vi "Dashboard Main.vi.REMOTE.11652.vi"() -> ()   [LabVIEW 2014]
uses:
  AutonModes.ctl
  <vilib>/event_ctls.llb/eventvkey.ctl
  <vilib>/Utility/error.llb/DialogType.ctl
  <vilib>/Rock Robotics/WPI/Dashboard/WPI_DashboardLogging Global.vi
  <vilib>/Rock Robotics/Network Tables/SD Write String.vi
  <vilib>/Rock Robotics/Network Tables/SD Read String.vi
  <vilib>/Utility/config.llb/Write Key (String).vi
  <vilib>/Utility/config.llb/Write Key (I32).vi
  <vilib>/Utility/config.llb/NI_LVConfig.lvlib
panel:
  in  "TCP":refnum<k5>
  in  "Rec Mode":enum32{"Stop", "Record", "Playback"}(radio)
  in  "Vision":u16(ring) items=["Camera Off", "USB Camera SW", "USB Camera HW", "IP Camera"]
  out "Camera IP":string
  out "Image Message":string="Timeout in Camera Communications"
  in  "Dashboard Tab":T1(tab)
  in  "Camera Settings":T2={"Frame Rate"=30, "Compression"=30, "Size"=1} {"Frame Rate" scale=1.0..30.0; "Size" items=["640x480", "320x240", "160x120"]}
  out "MotorChart R":cluster{"Numeric":dbl, "Numeric":dbl}(graph)
  out "MotorChart L":T3(graph)
  out "MotorSliders R":cluster{"MotorSlide1":dbl, "MotorSlide2":dbl} {"MotorSlide2" scale=-1.0..1.0 scale format="%#_2e"; "MotorSlide1" scale=-1.0..1.0 scale format="%#_2e"}
  out "MotorSliders L":T4 {"MotorSlide4 2" scale=0.0..14.0 scale format="%#_2e"; "MotorSlide2" scale=-1.0..1.0 scale format="%#_2e"; "MotorSlide1" scale=-1.0..1.0 scale format="%#_2e"}
  out "Gyro":dbl(knob) scale=0.0..360.0
  out "JS1 Z":dbl(slide) scale=-1.0..1.0 scale format="%#_2e"
  out "JS1 Graph":cluster{"X":dbl, "Y":dbl}[](graph)
  out "JS1 Buttons":T5
  out "JS2 Z":dbl(slide) scale=-1.0..1.0 scale format="%#_2e"
  out "JS2 Graph":cluster{"X":dbl, "Y":dbl}[](graph)
  out "JS2 Buttons":T5
  out "Mode":T6(ring)=enum."Auto Disabled"
  in  "DB Camera Config":bool
  out "fps":dbl format="%#.1g"
  out "Mbps":dbl format="%#.1g"
  out "Mbps 2":bool
  in  "Open Config File":bool
  in  "Auton Mode":T7
  in  "Path to Auton Configs":path=path "C:/AutoConfig"
  out "Current Overdraw":bool
  out "Current":T8(graph)
  in  "DB/String 9":string
  in  "DB/String 8":string
  in  "DB/String 7":string
  in  "DB/String 6":string
  in  "DB/String 5":string
  in  "DB/String 4":string
  in  "DB/String 3":string
  in  "DB/String 2":string
  in  "DB/String 1":string
  in  "DB/String 0":string
  in  "DB/Slider 0":dbl(slide) scale=0.0..5.0
  in  "DB/Slider 1":dbl(slide) scale=0.0..5.0
  in  "DB/Slider 2":dbl(slide) scale=0.0..5.0
  in  "DB/Slider 3":dbl(slide) scale=0.0..5.0
  out "DB/LED 3":bool
  out "DB/LED 2":bool
  out "DB/LED 1":bool
  out "DB/LED 0":bool
  in  "DB/Button 3":bool
  in  "DB/Button 2":bool
  in  "DB/Button 1":bool
  in  "DB/Button 0":bool caption="New Name"
  in  "Test Slider":dbl(slide) scale=0.0..100.0 scale format="%#_3g"
  in  "On/Off":bool caption="Solenoid"
  in  "Test Name":u16(ring) items=["Select the test to run...", "Example Test", "-------------------------------", "List of tests is built in robot code.", "Replace with your own automated tests."]
  in  "Test Tree":string(tree)
  in  "Motor":cluster{"Value":dbl, "Enable":bool} {"Value" scale=-1.0..1.0 scale format="%#_3g"}
  out "Progress":T9 {"Test Progress" scale=0.0..100.0}
  in  "Rev/Fwd":cluster{"Forward":bool, "Reverse":bool}
  in  "Test Ring":u16(ring) items=["Monochrome", "Color"]
  in  "Listbox":i32(listbox)
  out "Tree":string(tree)
  out "Camera Image":T10(plugin-control)
  out "Boolean":bool
  # "Left"
  # "Front"
  # "Right"
  # "Battery"
  # "This tab is a great place for autonomous settings and robot-specific values.\nPlace controls and indicators inside this tab and match name to\nDashboard Variables on robot. You can also delete this comment."
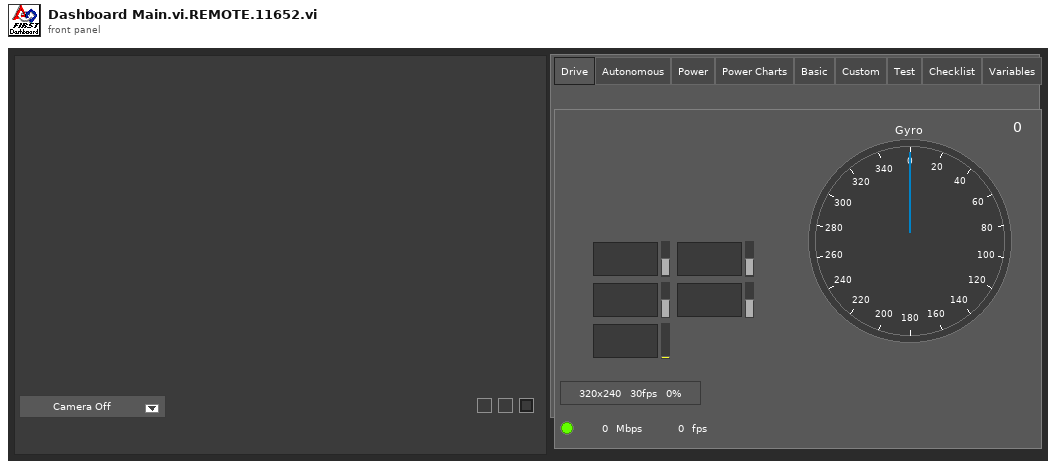
[diagram p1: front panel]
types:
  T1 = enum32{"Drive", "Autonomous", "Power", "Power Charts", "Basic", "Custom", "Test", "Checklist", "Variables"}
  T2 = cluster{"Frame Rate":i32, "Compression":i32, "Size":u16}
  T3 = cluster{"Numeric":dbl, "Numeric":dbl, "Battery V":dbl}
  T4 = cluster{"MotorSlide1":dbl, "MotorSlide2":dbl, "MotorSlide4 2":dbl}
  T5 = cluster{bool, bool, bool, bool, bool, bool, bool, bool, bool, bool, bool, bool}
  T6 = enum8{"Tele-Op Disabled", "Tele-Op Enabled", "Auto Disabled", "Auto Enabled", "Test Disabled", "Test Enabled", "Disconnected", "No Code", "E-Stop"}
  T7 = typedef "AutonModes.ctl" = enum32{"Sit Still", "Go Get That Tote!", "Custom 1", "Custom 2", "FromLandfill", "CanGrab"}
  T8 = cluster{"Numeric":dbl, "Numeric":dbl, "Numeric":dbl, "Numeric":dbl, "Numeric":dbl}
  T9 = cluster{"Test Progress":u8, "Test Progress Text":string}
  T10 = typedef "IMAQ Image.ctl" = refnum<image>
  T11 = enum32{"Drive", "Basic", "Custom", "Test", "Checklist", "Variables"}
  T12 = typedef "Image Type" = u32
  T13 = cluster{"Camera Image":refnum<vi>, "Dashboard Tab":refnum<vi>, "Boolean":refnum<vi>, "Vision":refnum<vi>, "Rec Mode":refnum<vi>, "Test Slider":refnum<vi>, "On/Off ":refnum<vi>, "Test Ring":refnum<vi>, "Rev/Fwd":refnum<vi>, "Test Name":refnum<vi>, "Motor":refnum<vi>, "Progress":refnum<vi>, "CheckList":refnum<vi>, "Tree":refnum<vi>, "Test Tree":refnum<vi>}
  T14 = enum16{"open", "replace", "create", "open or create", "replace or create", "replace or create with confirmation"}
  T15 = cluster{"Error Strings":string, "Disable Counts":cluster{u16, u16}, "Rail Faults":cluster{u16, u16, u16}, "Robot IP":string, "DB Mode":u8, "Event Info":cluster{"Name":string, "Type":u8, "Number":u16, "Replay":u8}, "Camera Addr":string}
  T16 = cluster{"Storage":cluster{"Disk Free":u64, "RAM Block":u32, "RAM free":u32}, "CPU Utilization":cluster{"CPU % ISR":sgl, "CPU % Time Crit":sgl, "CPU % Timed Str":sgl, "CPU % High":sgl, "CPU % Above":sgl, "CPU % Normal":sgl, "CPU % Low":sgl}, "CAN":cluster{"% Bus Utilization":sgl, "Bus Off Cnt":u32, "TX_FIFO Full Cnt":u32, "Receive Error Cnt":u8, "Transmit Error Cnt":u8}, "HID":cluster{"HID Outputs":u32, "Rumble Low":u16, "Rumble High":u16}[]}
  T17 = cluster{"Status bits":cluster{"Test Mode":bool, "Autonomous":bool, "Enabled":bool, "Code Start":bool, "Brownout":bool, "Reserved 2":bool, "Reserved 3":bool, "E-Stop":bool}, "Code Trace":cluster{"Disabled":bool, "TeleOp":bool, "Auto":bool, "Test":bool}, "Controller Type":enum16{"unknown", "cRIO", "roboRio"}, "Code?":enum16{"unknown", "noCode", "code"}, "Battery V":dbl}
  T18 = cluster{"Control Bits":cluster{"TestMode":bool, "Autonomous":bool, "Enabled":bool, "FMS Present":bool, bool, bool, bool, "E-Stop":bool}, "Team Station ":u8, "Countdown":sgl, "Joystick Values":cluster{"Axes":dbl[], "Buttons":bool[], "POVs":i16[]}[]}
  T19 = typedef "DialogType.ctl" = u16
  T20 = cluster{"Axes":dbl[], "Buttons":bool[], "POVs":i16[]}[]
  T21 = cluster{"Axes":dbl[], "Buttons":bool[], "POVs":i16[]}
  T22 = cluster{"Buttons[0]":bool, "Buttons[1]":bool, "Buttons[2]":bool, "Buttons[3]":bool, "Buttons[4]":bool, "Buttons[5]":bool, "Buttons[6]":bool, "Buttons[7]":bool, "Buttons[8]":bool, "Buttons[9]":bool, "Buttons[10]":bool, "Buttons[11]":bool}
  T23 = typedef "NI_LVConfig.lvlib/Config Data RefNum.ctl" = refnum<k1>
  T24 = cluster{"Operation":enum16{"Update", "Clear"}, "Color Box":u32}[]
  T25 = typedef "eventvkey.ctl" = enum16{"ASCII", "Enter", "Return", "Shift", "Ctrl", "Alt", "Cmd", "Opt", "Caps", "NumLock", "Clear", "Break", "Up", "Down", "Left", "Right", "Insert", "Delete", "Home", "End", "PageUp", "PageDown", "Escape", "Help", "Pause", "ScrollLock", "F1", "F2", "F3", "F4", "F5", "F6", "F7", "F8", "F9", "F10", "F11", "F12", "F13", "F14", "F15", "F16", "F17", "F18", "F19", "F20", "F21", "F22", "F23", "F24", "Play", "VolumeUp", "VolumeDown", "Mute", "Two Byte Char"}
  T26 = cluster{"Image Size":bool, "Image Type":bool, "Pixel Value":bool, "ROI Information":bool, "Zoom Factor":bool}
  T27 = enum8{"Enabled", "Disabled", "Disabled and Grayed Out"}
  T28 = cluster{"Operation":enum16{"Update", "Clear"}, "Color Box":u32}
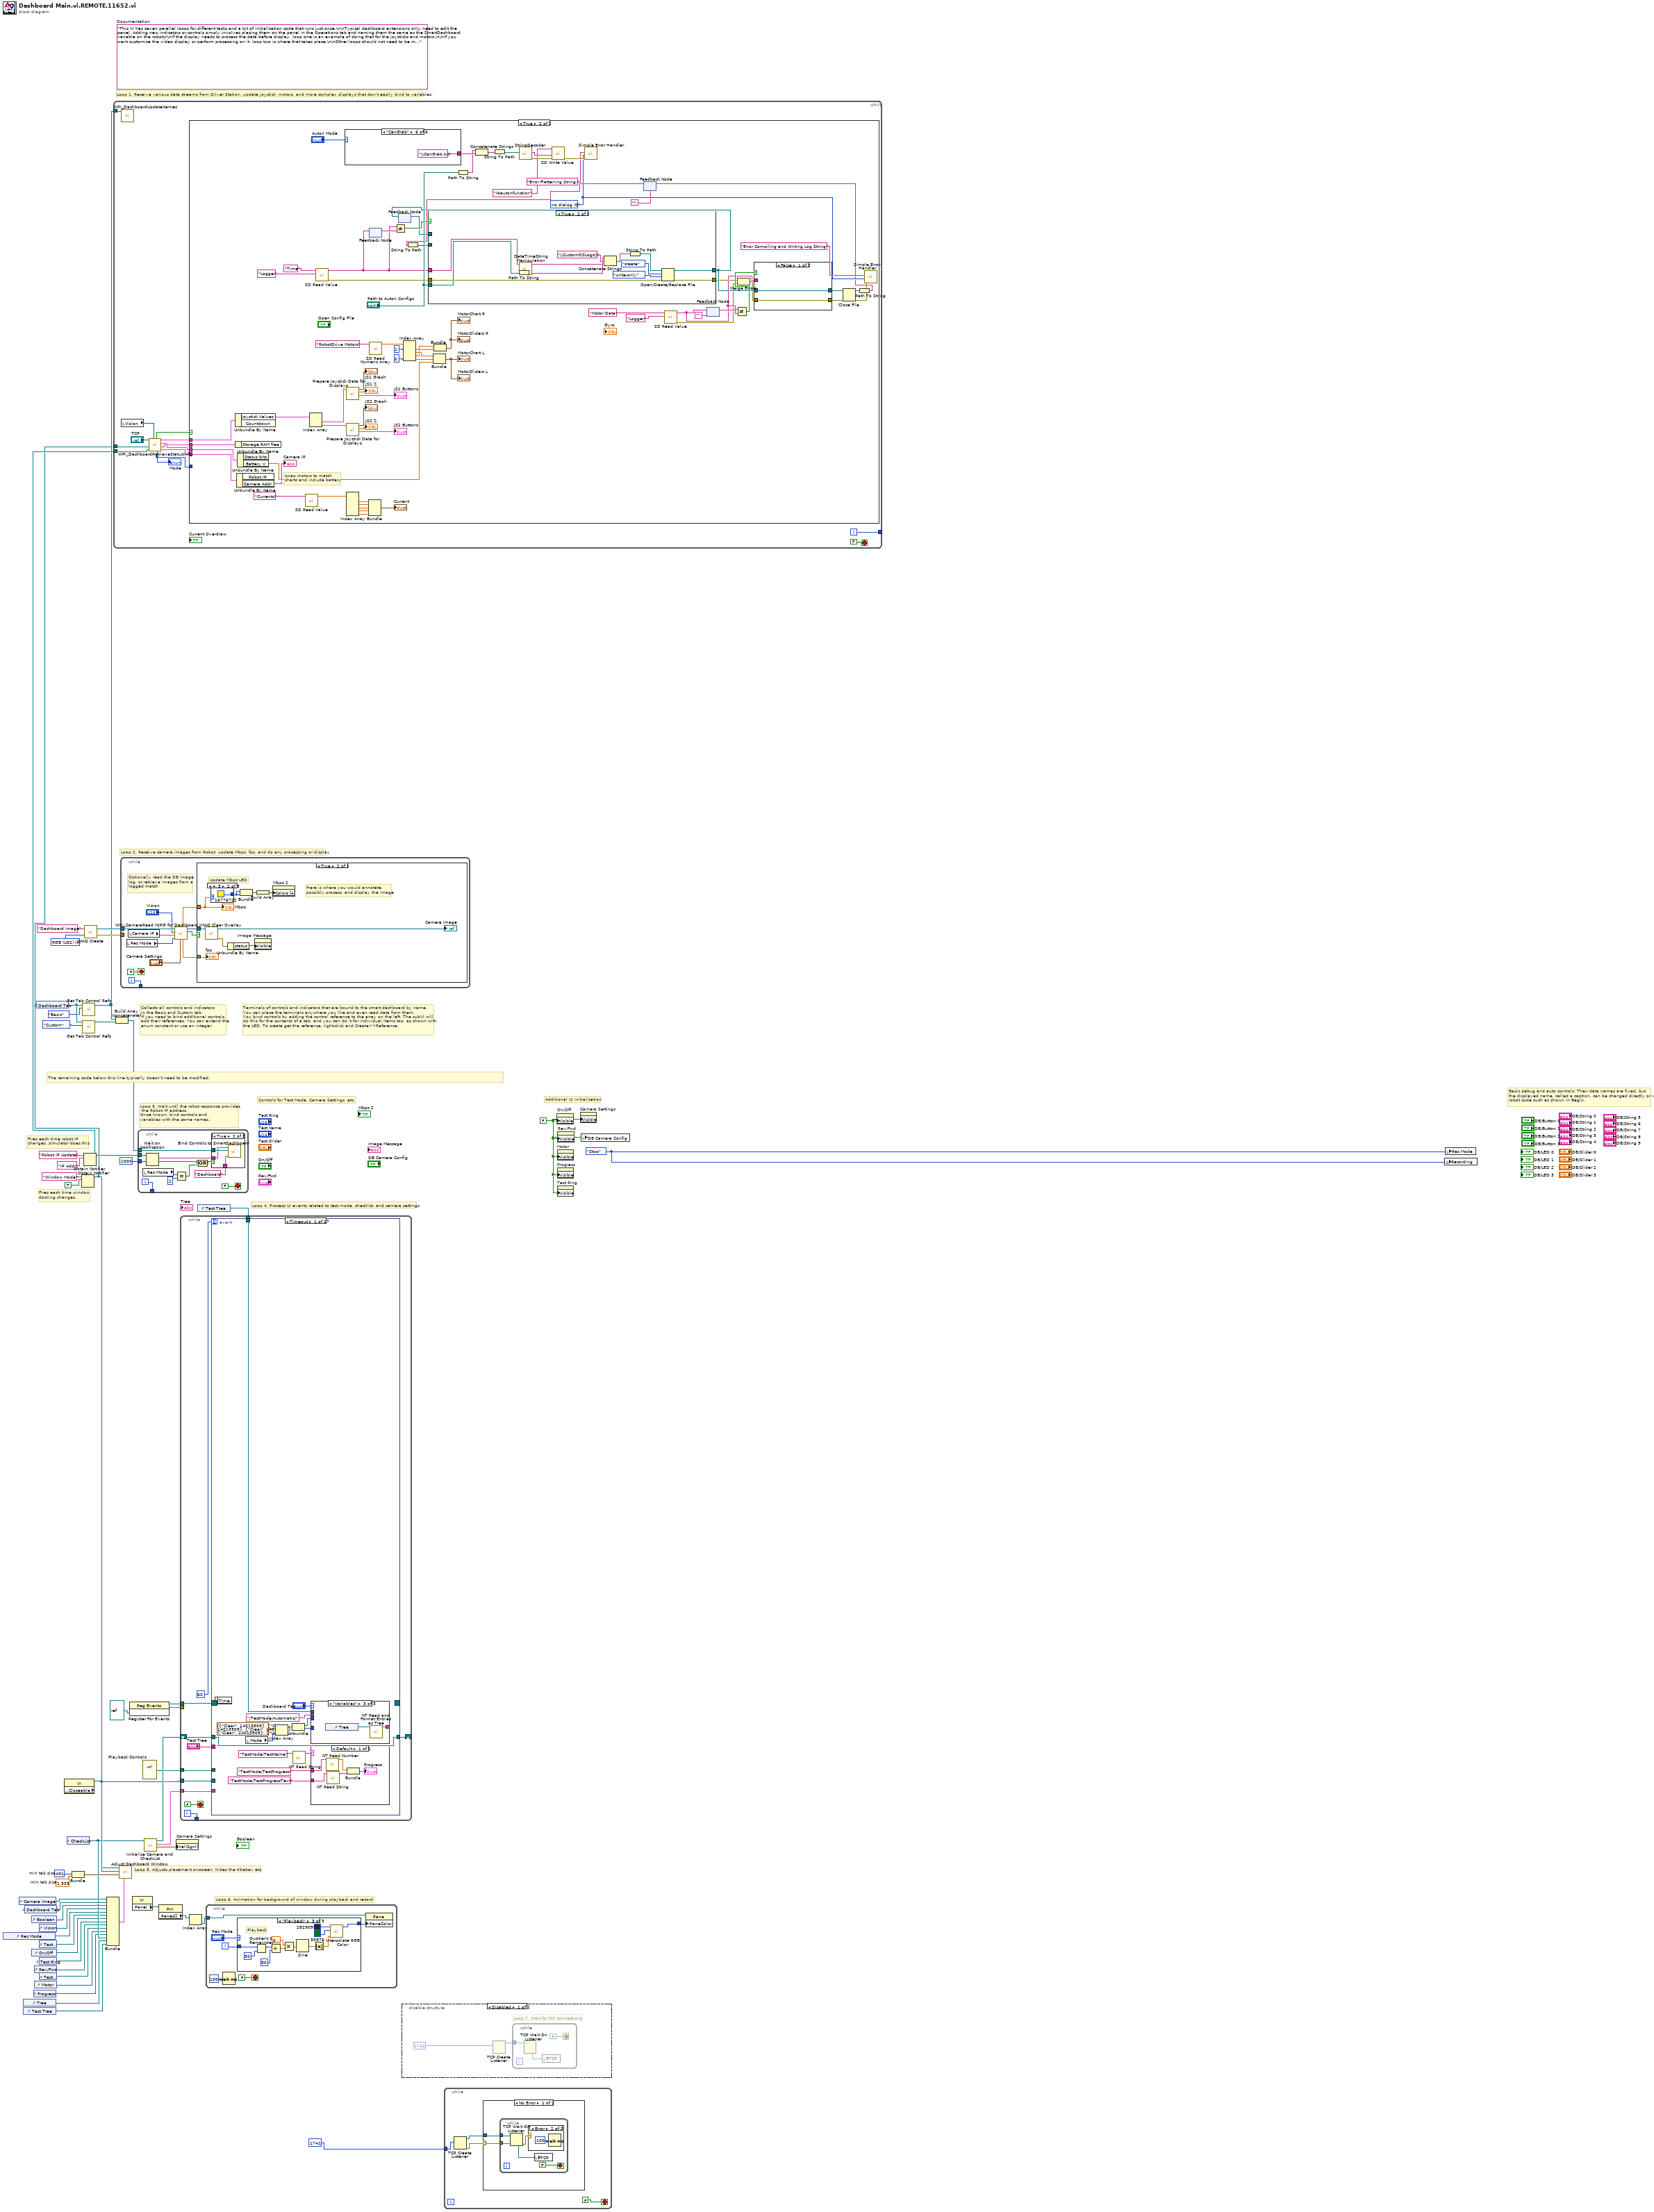
[diagram p0: block diagram]
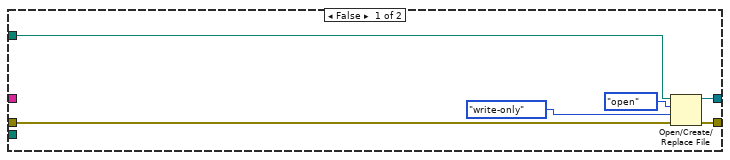
[diagram p6: hidden frame]
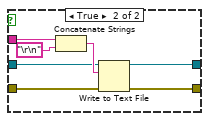
[diagram p7: hidden frame]
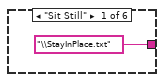
[diagram p8: hidden frame]
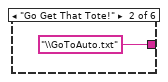
[diagram p9: hidden frame]
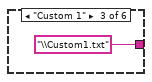
[diagram p10: hidden frame]
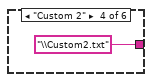
[diagram p11: hidden frame]
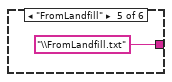
[diagram p12: hidden frame]
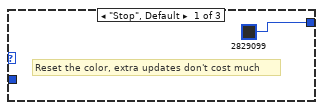
[diagram p13: hidden frame]
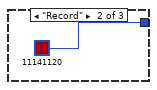
[diagram p14: hidden frame]
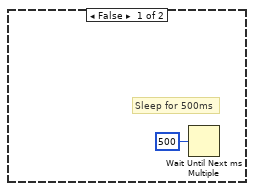
[diagram p16: hidden frame]
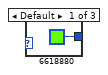
[diagram p17: hidden frame]
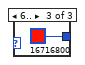
[diagram p18: hidden frame]
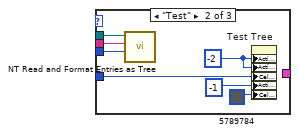
[diagram p20: hidden frame]
diagram:
  w23 = 491  # min tab size
  w22 = 1.333  # min tab size
  w31 = enum32{"Stop", "Record", "Playback"}."Stop" ("Rec Mode")
  w5 = FALSE ("Visible")
  (unwired) "This VI has seven parallel loops for different tasks and a bit of initialization code that runs just once.\n\nTypical dashboard extensions only need to edit the panel. Adding new indicators or controls simply involves placing them on the panel in the Operations tab and naming them the same as the SmartDashboard variable on the robot\n\nIf the display needs to process the data before display, loop one is an example of doing that for the joysticks and motors.\n\nIf you want customize the video display or perform processing on it, loop two is where that takes place.\n\nOther loops should not need to be modified. They are pretty standard, and document the task they perform."  # Documentation
  w51 = T12 4 items=["Grayscale (U8)", "Grayscale (I16)", "Grayscale (SGL)", "Complex (CSG)", "RGB (U32)", "HSL (U32)", "RGB (U64)"] ("Image Type")
  # "Basic debug and auto controls: Their data names are fixed, but\nthe displayed name, called a caption, can be changed directly or in\nrobot code such as shown in Begin."
  # "Controls for Test Mode, Camera Settings, etc."
  # "Additional UI Initialization"
  # "Loop 6. Animation for background of window during playback and record"
  # "Fires each time robot IP\nchanges, simulator does this"
  # "Fires each time window\ndocking changes."
  # "Collects all controls and indicators\nin the Basic and Custom tab.\nIf you need to bind additional controls,\nadd their references. You can extend the\nenum constant or use an integer."
  # "The remaining code below this line typically doesn't need to be modified."
  # "Loop 4. Process UI events related to test mode, checklist, and camera settings"
  # "Terminals of controls and indicators that are bound to the smart dashboard by name.\nYou can place the terminals anywhere you like and even read data from them.\nYou bind controls by adding the control reference to the array on the left. The subVI will\ndo this for the contents of a tab, and you can do it for individual items too, as shown with\nthe LED. To create get the reference, right-click and Create>>Reference."
  # "Loop 3. Wait until the robot response provides\n the Robot IP address.\nOnce known, bind controls and\nvariables with the same names."
  # "Loop 5. Adjusts placement onscreen, hides the titlebar, etc."
  # "Loop 1. Receive various data streams from Driver Station, update joystick, motors, and more complex displays that don't easily bind to variables."
  # "Loop 2. Receive camera images from Robot, update Mbps, fps, and do any processing or display"
  n1 = control-ref of="Rec Mode"() -> (w11:refnum<vi>)
  n2 = control-ref of="Camera Image"() -> (w26:refnum<vi>)
  n3 = control-ref of="Tree"() -> (w15:refnum<vi>)
  n4 = control-ref of="Test Tree"() -> (w14:refnum<vi>)
  n5 = control-ref of="Dashboard Tab"() -> (w25:refnum<vi>)
  n6 = control-ref of="Boolean"() -> (w20:refnum<vi>)
  n7 = control-ref of="On/Off"() -> (w9:refnum<vi>)
  n8 = control-ref of="Progress"() -> (w6:refnum<vi>)
  n9 = control-ref of="Rev/Fwd"() -> (w7:refnum<vi>)
  n10 = control-ref of="Motor"() -> (w12:refnum<vi>)
  n11 = control-ref of="Dashboard Tab"() -> (w29:refnum<vi>)
  n12 = control-ref of="Test Slider"() -> (w10:refnum<vi>)
  n13 = control-ref of="Vision"() -> (w24:refnum<vi>)
  n14 = control-ref of="Test Ring"() -> (w8:refnum<vi>)
  n15 = control-ref of="Test Name"() -> (w13:refnum<vi>)
  n16 = property class="VI" props=["Front Panel.Closeable"]() -> (reference out=w30:refnum<vi>)  [unwired: 2 in, 2 out]
  n17 = control-ref of="CheckList"() -> (w16:refnum<vi>)
  n18 = Bundle("min tab size"=w23, "min tab size"=w22) -> (w21:cluster{"min tab size":i32, "min tab size":dbl})  [unwired: 1 in]
  n19 = Obtain Notifier(name (unnamed)="Window Mode", notification data type=TRUE) -> (notifier out=w2:refnum<notifier>)  [unwired: 2 in, 2 out]
  n20 = call <vilib>:"Get Tab Control Refs.vi"("Page Index"=T11."Basic" ("Dashboard Tab"), "TabControl in"=w29) -> ("ControlsOnPage"=w3:refnum<vi>[])  [unwired: 9 in]
  n21 = call <vilib>:"Get Tab Control Refs.vi"("Page Index"=T11."Custom" ("Dashboard Tab"), "TabControl in"=w29) -> ("ControlsOnPage"=w28:refnum<vi>[])  [unwired: 9 in]
  n22 = Obtain Notifier(name (unnamed)="Robot IP Update", notification data type="IP Addr" ("name (unnamed)")) -> (notifier out=w4:refnum<notifier>)  [unwired: 2 in, 2 out]
  n23 = call "IMAQ Create"("Image Name"="Dashboard Image", "Image Type"=w51) -> ("New Image"=w49:T10, "error out"=w48:errorcluster)  [unwired: 2 in, 1 out]
  n24 = Bundle("Camera Image"=w26, "Dashboard Tab"=w25, "Boolean"=w20, "Vision"=w24, "Rec Mode"=w11, "Test Slider"=w10, "On/Off"=w9, "Test Ring"=w8, "Rev/Fwd"=w7, "Test Name"=w13, "Motor"=w12, "Progress"=w6, "CheckList"=w16, "Tree"=w15, "Test Tree"=w14) -> (w17:T13)  [unwired: 1 in]
  n25 = while {
    tunnel: [w63] -> _
    tunnel: w4 -> [w57]
    tunnel: w3 -> [w56]
    tunnel: w2 -> [w52]
    i -> [w63]
    stop <- FALSE stop-if-true
    n26 = call <vilib>:"WPI_DashboardUpdateNames.vi"("Controls on Tab"=w56) -> ()  [unwired: 11 in]
    n27 = local read "Vision"() -> (w54:u16)
    n28 = call <vilib>:"WPI_DashboardRetrieveStatusInfo.vi"("Vision"=w54, "Binding Refnum"=w57, "Window Mode Notifier"=w52, "TCP Cnx"="TCP") -> ("Power and Errors"=w58:T15, "Robot Metrics"=w61:T16, "Status Info"=w62:T17, "Control Info"=w59:T18, "Robot Mode"=w55:T6, "Process?"=w60:bool)  [unwired: 2 in]
    "Mode" <- w55
    n29 = case shown="True" w60 {
      tunnel: w62 -> [_ w135]
      tunnel: w61 -> [_ w134]
      tunnel: w59 -> [_ w133]
      tunnel: w58 -> [_ w132]
      tunnel: w55 -> [_ _]
      frame False {
      }
      frame True {
        w75 = T19 0 items=["no dialog", "OK message", "continue or stop message", "OK message + warnings", "continue/stop + warnings"] ("type of dialog (OK msg:1)")
        # "swap motors to match\ncharts and include battery"
        n30 = Unbundle By Name(w133) -> ("Joystick Values"=w120:T20)  [unwired: 1 out]
        n31 = Unbundle By Name(w134) -> ()  [unwired: 1 out]
        n32 = Unbundle By Name(w132) -> ("Camera Addr"=→"Camera IP":string)  [unwired: 1 out]
        n33 = Unbundle By Name(w135) -> ("Battery V"=w121:dbl)  [unwired: 1 out]
        n34 = call-poly <vilib>:"SD Read Value.vi"("Name"="Currents") -> ("Numeric Array"=w106:dbl[])  [unwired: 8 in, 2 out]
        n35 = Index Array(array=w120) -> (element #1=w119:T21, element #2=w114:T21)  [unwired: 2 in]
        n36 = call-poly <vilib>:"SD Read Value.vi"("Table Prefix"="Logger", "Name"="Time") -> ("error out"=w76:errorcluster, "String"=w84:string)  [unwired: 7 in, 1 out]
        n37 = case shown="\"CanGrab\"" "Auton Mode" {
          tunnel: ["\\StayInPlace.txt" "\\GoToAuto.txt" "\\Custom1.txt" "\\Custom2.txt" "\\FromLandfill.txt" "\\CanGrab.txt"] -> w99
          frame "Sit Still" {
          }
          frame "Go Get That Tote!" {
          }
          frame "Custom 1" {
          }
          frame "Custom 2" {
          }
          frame "FromLandfill" {
          }
          frame "CanGrab" {
          }
        }
        n38 = call "Prepare Joystick Data for Displays.vi"("Joystick Values"=w119) -> ("Buttons"=→"JS1 Buttons":T22, "Z Axis"=→"JS1 Z":dbl, "Cartesian Data"=→"JS1 Graph":cluster{"X axis":dbl, "X axis":dbl}[])  [unwired: 8 in]
        n39 = call "Prepare Joystick Data for Displays.vi"("Joystick Values"=w114) -> ("Buttons"=→"JS2 Buttons":T22, "Z Axis"=→"JS2 Z":dbl, "Cartesian Data"=→"JS2 Graph":cluster{"X axis":dbl, "X axis":dbl}[])  [unwired: 8 in]
        n40 = Index Array(array=w106) -> (element #1=w105:dbl, element #2=w104:dbl, element #3=w103:dbl, element #4=w102:dbl, element #5=w101:dbl)  [unwired: 5 in]
        n41 = Bundle("Numeric"=w105, "Numeric"=w104, "Numeric"=w103, "Numeric"=w102, "Numeric"=w101) -> (→"Current":T8)  [unwired: 1 in]
        n42 = feedback #1() -> (w86:string)  [unwired: 1 in]
        n43 = feedback-in #1(w84) -> ()
        n44 = call <vilib>:"SD Read Numeric Array.vi"("Name"="RobotDrive Motors") -> ("Numeric Array"=w123:dbl[])  [unwired: 8 in, 2 out]
        n45 = Not Equal?(x=w84, y=w86) -> (x != y?=w85:bool)
        n46 = feedback #2() -> (w83:refnum<file>)  [unwired: 1 in]
        n47 = Index Array(array=w123, index #1=1, index #4=0) -> (element #1=w127:dbl, element #2=w128:dbl, element #3=w126:dbl, element #4=w131:dbl)  [unwired: 2 in]
        n48 = Bundle("Numeric"=w128, "Numeric"=w131, "Battery V"=w121) -> (→"MotorChart L" →"MotorSliders L":T3)  [unwired: 1 in]
        n49 = Bundle("Numeric"=w126, "Numeric"=w127) -> (→"MotorChart R" →"MotorSliders R":cluster{"Numeric":dbl, "Numeric":dbl})  [unwired: 1 in]
        n50 = Path To String(path="Path to Auton Configs") -> (string=w98:string)
        n51 = Concatenate Strings(w98, w99) -> (w97:string)
        n52 = String To Path(string=w97) -> (path=w96:path)
        n53 = call "StringDecoder.vi"("Auto Config File"=w96) -> ("error out"=w81:errorcluster, "RobotDataString"=w109:string)  [unwired: 9 in]
        n54 = call-poly <vilib>:"SD Write Value.vi"("error in"=w81, "String"=w109, "Name"="rbautonfunction") -> ("error out"=w80:errorcluster)  [unwired: 7 in, 1 out]
        n55 = call <vilib>:"Simple Error Handler.vi"("error source (\" \")"="Error Flattening String:", "type of dialog (OK msg:1)"=w75, "error in (no error)"=w80) -> ()  [unwired: 2 in, 5 out]
        n56 = feedback #3("") -> (w65:string)
        n57 = String To Path(string=w65) -> (path=w68:path)
        n58 = case shown="True" w85 {
          tunnel: "Path to Auton Configs" -> [_ w150]
          tunnel: w84 -> [_ w151]
          tunnel: [w141 w152] -> w82
          tunnel: w83 -> [_ _]
          tunnel: w76 -> [w138 w142]
          tunnel: [w137 w149] -> w79
          tunnel: w68 -> [w136 _]
          frame False {
            n59 = Open/Create/Replace File(file path (use dialog)=w136, error in=w138, operation (0:open)=T14."open", access (0:read/write)=enum16{"read/write", "read-only", "write-only"}."write-only") -> (refnum out=w141:refnum<file>, error out=w137:errorcluster)  [unwired: 2 in, 1 out]
          }
          frame True {
            n60 = Path To String(path=w150) -> (string=w146:string)
            n61 = call "DateTimeString Manipulation.vi"("FPU DT String"=w151) -> ("FPF DT String"=w144:string)  [unwired: 4 in]
            n62 = Concatenate Strings(w146, "\\CustomDSLogs\\", w144) -> (w147:string)
            n63 = String To Path(string=w147) -> (path=w153:path)
            n64 = Open/Create/Replace File(file path (use dialog)=w153, error in=w142, operation (0:open)=T14."create", access (0:read/write)=enum16{"read/write", "read-only", "write-only"}."write-only") -> (refnum out=w152:refnum<file>, error out=w149:errorcluster)  [unwired: 2 in, 1 out]
          }
        }
        n65 = feedback-in #2(w82) -> ()
        n66 = call-poly <vilib>:"SD Read Value.vi"("Table Prefix"="Logger", "Name"="Motor Data") -> ("error out"=w78:errorcluster, "String"=w90:string)  [unwired: 7 in, 1 out]
        n67 = feedback-in #4(w90) -> ()
        n68 = feedback #4("") -> (w92:string)
        n69 = Not Equal?(x=w90, y=w92) -> (x != y?=w91:bool)
        n70 = Merge Errors(w79, w78) -> (w77:errorcluster)
        n71 = case shown="False" w91 {
          tunnel: w90 -> [_ w161]
          tunnel: w82 -> [w154 w159]
          tunnel: w77 -> [w155 w158]
          tunnel: [w155 w157] -> w72
          tunnel: [w154 w156] -> w70
          frame False {
          }
          frame True {
            n72 = Concatenate Strings(w161, "\r\n") -> (w160:string)
            n73 = Write to Text File(file (use dialog)=w159, text=w160, error in=w158) -> (refnum out=w156:refnum<file>, error out=w157:errorcluster)  [unwired: 1 in, 1 out]
          }
        }
        n74 = Close File(refnum=w70, error in=w72) -> (path=w67:path, error out=w71:errorcluster)
        n75 = Path To String(path=w67) -> (string=w66:string)
        n76 = feedback-in #3(w66) -> ()
        n77 = call <vilib>:"Simple Error Handler.vi"("error source (\" \")"="Error Compiling and Writing Log String", "type of dialog (OK msg:1)"=w75, "error in (no error)"=w71) -> ()  [unwired: 2 in, 5 out]
      }
    }
  }
  n78 = Build Array (concatenate)(w3, w28) -> (w27:refnum<vi>[])
  n79 = call "Adjust Dashboard Window.vi"("Sizing Refnums"=w17, "Size Constraints"=w21, "VI"=w30, "Notifier in"=w2) -> ()  [unwired: 8 in]
  n80 = while {
    tunnel: w49 -> [w177]
    tunnel: w48 -> [_]
    tunnel: [w178] -> _
    i -> [w178]
    stop <- FALSE stop-if-true
    # "Optionally read the DB image,\nlog, or retrieve images from a\nlogged match"
    n81 = local read "Rec Mode"() -> (w171:enum32{"Stop", "Record", "Playback"})
    n82 = local read "Camera IP"() -> (w169:string)
    n83 = call <vilib>:"WPI_CameraRead MJPG for Dashboard.vi"("Camera Settings"="Camera Settings", "Rec Mode"=w171, "Camera IP"=w169, "Camera Mode"="Vision", "Refnum in"=w177) -> ("Active"=w175:bool, "Refnum out"=w176:T10, "FPS"=w174:dbl, "Bandwidth (Mbps)"=w173:dbl)  [unwired: 3 in]
    n84 = case shown="True" w175 {
      tunnel: w176 -> [_ w184]
      tunnel: w173 -> [_ w183]
      tunnel: w174 -> [_ w181]
      frame False {
        # "Sleep for 500ms"
        n85 = Wait Until Next ms Multiple(millisecond multiple=u32 500) -> ()  [unwired: 1 out]
      }
      frame True {
        # "Here is where you would annotate,\npossibly process, and display the image"
        # "Update Mbps LED"
        n86 = call "IMAQ Clear Overlay"("Image"=w184) -> ("error out"=w188:errorcluster, "Image Out"=→"Camera Image":T10)  [unwired: 2 in, 7 out]
        n87 = case shown="4, 5" w183 {
          tunnel: [u32 6618880 ("Color Box") u32 16776722 ("Color Box") u32 16716800 ("Color Box")] -> w185
          frame Default {
          }
          frame 4, 5 {
          }
          frame 6.. {
          }
        }
        n88 = Unbundle By Name(w188) -> ("status"=w189:bool)
        n89 = Bundle("Color Box"=w185, "Color Box"=w185) -> (w187:cluster{"Color Box":u32, "Color Box":u32})  [unwired: 1 out]
        n90 = property on="Image Message" class="Str"("Visible"=w189) -> ()  [unwired: 2 in, 2 out]
        n91 = Build Array(w187) -> (w186:cluster{"Color Box":u32, "Color Box":u32}[])
        n92 = property on="Mbps 2" class="Bool (strict)"("Colors [4]"=w186) -> ()  [unwired: 2 in, 2 out]
        "Mbps" <- w183
        "fps" <- w181
      }
    }
  }
  n93 = register-events(refnum<vi> refnum) -> (reference out=w35:refnum<event-registration>, error out=w34:errorcluster)  [unwired: 2 in]
  n94 = property class="VI"() -> ("Panel"=w38:refnum<vi>)  [unwired: 2 in, 2 out]
  n95 = while {
    tunnel: w27 -> [w204]
    tunnel: w4 -> [w202]
    tunnel: [w200] -> _
    tunnel: u32 1000 ("milliseconds to wait") -> [w199]
    i -> [w200]
    stop <- FALSE stop-if-true
    n96 = local read "Rec Mode"() -> (w195:enum32{"Stop", "Record", "Playback"})
    n97 = Wait on Notification(notifier=w202, timeout in ms (-1)=w199) -> (notification=w201:string, timed out?=w197:bool)  [unwired: 2 in, 2 out]
    n98 = Equal?(x=w195, y=u16 2 ("Rec Mode")) -> (x = y?=w196:bool)
    n99 = Compound Arithmetic op=OR(invert w197, w196) -> (w198:bool)
    n100 = case shown="True" w198 {
      tunnel: w204 -> [_ w207]
      tunnel: w201 -> [_ w206]
      tunnel: "Dashboard" -> [_ w205]
      frame False {
      }
      frame True {
        n101 = call <vilib>:"Bind Controls to SmartDashboard.vi"("Client Name"=w205, "Bound Control Refs"=w207, "Server IP Address"=w206) -> ()  [unwired: 9 in]
      }
    }
  }
  n102 = vi-ref "Playback Controls.vi"() -> (w36:refnum<vi>)
  n103 = call "Initialize Camera and CheckList.vi"("ListBox in"=w16) -> ("Cluster"=w42:cluster{"value":i32, "value":i32, "index":i32}, "Array"=w43:cluster{string[]}[], "File Refnum"=w41:T23)  [unwired: 8 in]
  n104 = property class="Pnl"(reference=w38) -> ("Panes[]"=w39:refnum<vi>[])  [unwired: 1 in, 2 out]
  n105 = property on="Camera Settings" class="Clust (strict)"("Val(Sgnl)"=w42) -> ()  [unwired: 2 in, 2 out]
  n106 = Index Array(array=w39) -> (element=w37:refnum<vi>)  [unwired: 1 in]
  n107 = control-ref of="Test Tree"() -> (w40:refnum<vi>)
  n108 = while {
    tunnel: w43 -> [w215]
    shift-right: [w214] -> _
    shift-left: w41 -> [w213]
    tunnel: [w212] -> _
    tunnel: w40 -> [w211]
    tunnel: w36 -> [w210]
    tunnel: w35 -> [w209]
    tunnel: w34 -> [_]
    tunnel: w30 -> [w208]
    i -> [w212]
    stop <- FALSE stop-if-true
    n109 = event shown="[0] Timeout" {
      selector: w209 -> [_ _ _ _ _ _ _ _ _ _ _ _ _ _ _ _ _]
      dyn-events: [_ _ _ _ _ _ _ _ _ _ _ _ _ w453 _ _ _] -> _
      timeout: u32 60 ("milliseconds to wait") -> [_ _ _ _ _ _ _ _ _ _ _ _ _ _ _ _ _]
      tunnel: w211 -> [w227 _ _ _ _ _ _ _ _ _ _ _ _ _ _ _ _]
      tunnel: "Test Tree" -> [_ _ _ _ _ _ _ _ w422 w430 w432 w436 w444 _ _ _ _]
      tunnel: w215 -> [_ w249 _ _ _ _ w386 w416 _ _ _ _ _ _ _ _ _]
      tunnel: [w223 w248 w347 w352 w360 w372 w385 w409 w421 w428 w431 w435 w443 w455 w469 w470 w480] -> w214
      tunnel: w213 -> [w223 w248 w347 w352 w360 w372 w384 w409 w421 w428 w431 w435 w443 w455 w469 w470 w480]
      tunnel: w210 -> [_ _ _ _ _ _ _ _ _ _ _ _ _ w456 _ w473 _]
      tunnel: w208 -> [_ _ _ _ _ _ _ _ _ _ _ _ _ w451 _ _ _]
      event Timeout {
        n110 = event-data() -> ()  [unwired: 1 in, 1 out]
        n111 = local read "Mode"() -> (w226:T6)
        n112 = Index Array(array=T24 [{"Operation"=enum."Clear", "Color Box"=14013909}, {"Operation"=enum."Clear", "Color Box"=14013909}, {"Operation"=enum."Clear", "Color Box"=14013909}, {"Operation"=enum."Clear", "Color Box"=14013909}, {"Operation"=enum."Update", "Color Box"=14013909}, {"Operation"=enum."Update", "Color Box"=16777215}, {"Operation"=enum."Clear", "Color Box"=14013909}, {"Operation"=enum."Clear", "Color Box"=14013909}, {"Operation"=enum."Clear", "Color Box"=14013909}], index=w226) -> (element=w221:T28)
        n113 = Unbundle(w221) -> ("Operation"=w220:enum16{"Update", "Clear"}, "Color Box"=w219:u32)
        n114 = call <vilib>:"NT Read String.vi"("Name"="TestMode/TestName") -> ("String"=w230:string)  [unwired: 9 in, 1 out]
        n115 = case shown="\"Variables\"" "Dashboard Tab" {
          tunnel: w227 -> [_ w238 _]
          tunnel: "/TestMode/Automatic/" ("Name Pattern") -> [_ w237 _]
          tunnel: w220 -> [_ w236 _]
          tunnel: [_ _ w240] -> _
          tunnel: w219 -> [_ w232 _]
          frame "Custom", Default {
          }
          frame "Test" {
            w235 = -2 ("Active Item:Row Number")
            n116 = call <vilib>:"NT Read and Format Entries as Tree.vi"("Operation"=w236, "Name Pattern"=w237, "Tree Refnum"=w238) -> ()  [unwired: 7 in, 2 out]
            n117 = property on="Test Tree" class="Tree (strict)"("Active Item Row Number"=w235, "ActiveColNum"=w235, "CellBG"=w232, "Active Item Row Number"=-1 ("Active Item:Row Number"), "CellBG"=u32 5789784 ("Color Box")) -> ()  [unwired: 2 in, 2 out]
          }
          frame "Variables" {
            n118 = control-ref of="Tree"() -> (w239:refnum<vi>)
            n119 = call <vilib>:"NT Read and Format Entries as Tree.vi"("Tree Refnum"=w239) -> ("Formatted Strings"=w240:cluster{"Name":string, "Value":string}[])  [unwired: 9 in, 1 out]
          }
        }
        n120 = case shown="Default" w230 {
          tunnel: "TestMode/TestProgress" ("Name") -> [w242 _]
          tunnel: "TestMode/TestProgressText" ("Name") -> [w241 _]
          frame Default {
            n121 = call <vilib>:"NT Read Number.vi"("Name"=w242) -> ("Numeric"=w243:dbl)  [unwired: 9 in, 1 out]
            n122 = call <vilib>:"NT Read String.vi"("Name"=w241) -> ("String"=w244:string)  [unwired: 9 in, 1 out]
            n123 = Bundle("Numeric"=w243, "String"=w244) -> (→"Progress":cluster{"Numeric":dbl, "String":string})  [unwired: 1 in]
          }
          frame "" {
            n124 = property on="Progress" class="Clust (strict)"("Visible"=FALSE) -> ()  [unwired: 2 in, 2 out]
            n125 = local write "Test Name"(u16 0) -> ()
          }
        }
      }
      event "Test Tree": Value Change {
        # "Show appropriate\ncontrols"
        n126 = event-data() -> ("CtlRef"=w252:refnum<vi>, "NewVal"=w250:string)  [unwired: 1 in]
        n127 = call <vilib>:"WPI_UtilitiesGetTreeIOName.vi"("NewVal"=w250, "TreeControl in"=w252) -> ("I/O Name"=w253:string)  [unwired: 9 in]
        n128 = case shown="\"Camera\"" w253 {
          selector: w253 -> [_ w260 _ w278 w287 _]
          tunnel: w250 -> [_ _ w275 w277 _ w294]
          tunnel: w249 -> [_ _ _ _ _ w293]
          frame Default {
            w255 = FALSE ("Visible")
            w254 = FALSE ("Visible")
            n129 = property on="Motor" class="Clust (strict)"("Visible"=w254) -> ()  [unwired: 2 in, 2 out]
            n130 = property on="Test Ring" class="Ring (strict)"("Visible"=w254) -> ()  [unwired: 2 in, 2 out]
            n131 = property on="Rev/Fwd" class="Clust (strict)"("Visible"=w255) -> ()  [unwired: 2 in, 2 out]
            n132 = property on="On/Off" class="Bool (strict)"("Visible"=w255) -> ()  [unwired: 2 in, 2 out]
            n133 = property on="Test Slider" class="Slide (strict)"("Visible"=w255) -> ()  [unwired: 2 in, 2 out]
          }
          frame "Motor", "PWM" {
            w261 = FALSE ("Visible")
            n134 = case shown="\"Motor\", Default" w260 {
              tunnel: [1.0 ("Value") -1.0 ("Value")] -> w259
              tunnel: [255.0 ("Value") 1.0 ("Value")] -> w258
              tunnel: [128.0 ("Value") 0.0 ("Value")] -> w257
              tunnel: [64.0 ("Value") 0.5 ("Value")] -> w256
              frame "PWM" {
              }
              frame "Motor", Default {
              }
            }
            n135 = property on="Motor" class="Clust (strict)"("Visible"=TRUE) -> ()  [unwired: 2 in, 2 out]
            n136 = property on="Value" class="Slide (strict)"("Value"=w257, "Scale.Minimum"=w259, "Scale.Maximum"=w258, "Scale.Increment"=w256) -> ()  [unwired: 2 in, 2 out]
            n137 = property on="On/Off" class="Bool (strict)"("Visible"=w261) -> ()  [unwired: 2 in, 2 out]
            n138 = property on="Test Slider" class="Slide (strict)"("Visible"=w261) -> ()  [unwired: 2 in, 2 out]
            n139 = property on="Test Ring" class="Ring (strict)"("Visible"=w261) -> ()  [unwired: 2 in, 2 out]
            n140 = property on="Rev/Fwd" class="Clust (strict)"("Visible"=w261) -> ()  [unwired: 2 in, 2 out]
          }
          frame "Servo" {
            w273 = FALSE ("Visible")
            n141 = call <vilib>:"NT Read Number.vi"("Name"=w275) -> ("Numeric"=w274:dbl)  [unwired: 9 in, 1 out]
            n142 = property on="Test Slider" class="Slide (strict)"("Visible"=TRUE, "Scale.Maximum"=170.0 ("Scale.Range:Maximum")) -> ()  [unwired: 2 in, 2 out]
            n143 = local write "Test Slider"(w274) -> ()
            n144 = property on="Motor" class="Clust (strict)"("Visible"=w273) -> ()  [unwired: 2 in, 2 out]
            n145 = property on="Rev/Fwd" class="Clust (strict)"("Visible"=w273) -> ()  [unwired: 2 in, 2 out]
            n146 = property on="On/Off" class="Bool (strict)"("Visible"=w273) -> ()  [unwired: 2 in, 2 out]
            n147 = property on="Test Ring" class="Ring (strict)"("Visible"=w273) -> ()  [unwired: 2 in, 2 out]
          }
          frame "Relay", "Solenoid" {
            w276 = FALSE ("Visible")
            n148 = property on="Motor" class="Clust (strict)"("Visible"=w276) -> ()  [unwired: 2 in, 2 out]
            n149 = property on="Test Slider" class="Slide (strict)"("Visible"=w276) -> ()  [unwired: 2 in, 2 out]
            n150 = Search and Replace String(input string=w277, search string="/Value  **", replace string="/Direction") -> (result string=w283:string)  [unwired: 5 in, 3 out]
            n151 = property on="Test Ring" class="Ring (strict)"("Visible"=w276) -> ()  [unwired: 2 in, 2 out]
            n152 = call <vilib>:"NT Read String.vi"("Name"=w283) -> ("String"=w281:string)  [unwired: 9 in, 1 out]
            n153 = Equal?(x="Both directions", y=w281) -> (x = y?=w279:bool)
            n154 = Not(x=w279) -> (.not. x?=w280:bool)
            n155 = property on="Rev/Fwd" class="Clust (strict)"("Visible"=w279) -> ()  [unwired: 2 in, 2 out]
            n156 = property on="On/Off" class="Bool (strict)"("Visible"=w280, "Caption.Text"=w278) -> ()  [unwired: 2 in, 2 out]
          }
          frame "Compressor", "Digital Out" {
            w286 = FALSE ("Visible")
            # "Get direction and finish"
            n157 = property on="Motor" class="Clust (strict)"("Visible"=w286) -> ()  [unwired: 2 in, 2 out]
            n158 = property on="Test Slider" class="Slide (strict)"("Visible"=w286) -> ()  [unwired: 2 in, 2 out]
            n159 = property on="Test Ring" class="Ring (strict)"("Visible"=w286) -> ()  [unwired: 2 in, 2 out]
            n160 = property on="On/Off" class="Bool (strict)"("Visible"=TRUE, "Caption.Text"=w287) -> ()  [unwired: 2 in, 2 out]
            n161 = property on="Rev/Fwd" class="Clust (strict)"("Visible"=FALSE) -> ()  [unwired: 2 in, 2 out]
          }
          frame "Camera" {
            n162 = call <vilib>:"Get Last Path Segment.vi"("String in"=w294) -> ("String out"=w295:string)  [unwired: 10 in]
            n163 = property on="On/Off" class="Bool (strict)"("Visible"=FALSE) -> ()  [unwired: 2 in, 2 out]
            n164 = property on="Motor" class="Clust (strict)"("Visible"=FALSE) -> ()  [unwired: 2 in, 2 out]
            n165 = property on="Rev/Fwd" class="Clust (strict)"("Visible"=FALSE) -> ()  [unwired: 2 in, 2 out]
            n166 = case shown="\"White Balance  **\"" w295 {
              tunnel: w294 -> [w301 w310 w319 w328 w337 _ w343]
              tunnel: w293 -> [w299 w307 w316 w325 w334 _ _]
              frame "Size  **" {
                n167 = Index Array(array=w299) -> (element=w298:cluster{string[]})  [unwired: 1 in]
                n168 = call <vilib>:"NT Read String.vi"("Name"=w301) -> ("String"=w300:string)  [unwired: 9 in, 1 out]
                n169 = Unbundle(w298) -> (w296:string[])
                n170 = Match First String(2:w296, 3:w300) -> (0:w297:i32)  [unwired: 1 out]
                n171 = property on="Test Ring" class="Ring (strict)"("Value"=w297, "Strings []"=w296) -> ()  [unwired: 2 in, 2 out]
                n172 = property on="Test Ring" class="Ring (strict)"("Visible"=TRUE) -> ()  [unwired: 2 in, 2 out]
                n173 = property on="Test Slider" class="Slide (strict)"("Visible"=FALSE) -> ()  [unwired: 2 in, 2 out]
              }
              frame "White Balance  **" {
                n174 = Index Array(array=w307, index=1) -> (element=w308:cluster{string[]})
                n175 = call <vilib>:"NT Read String.vi"("Name"=w310) -> ("String"=w309:string)  [unwired: 9 in, 1 out]
                n176 = Unbundle(w308) -> (w305:string[])
                n177 = Match First String(2:w305, 3:w309) -> (0:w304:i32)  [unwired: 1 out]
                n178 = property on="Test Ring" class="Ring (strict)"("Value"=w304, "Strings []"=w305) -> ()  [unwired: 2 in, 2 out]
                n179 = property on="Test Ring" class="Ring (strict)"("Visible"=TRUE) -> ()  [unwired: 2 in, 2 out]
                n180 = property on="Test Slider" class="Slide (strict)"("Visible"=FALSE) -> ()  [unwired: 2 in, 2 out]
              }
              frame "Exposure  **" {
                n181 = Index Array(array=w316, index=2) -> (element=w317:cluster{string[]})
                n182 = call <vilib>:"NT Read String.vi"("Name"=w319) -> ("String"=w318:string)  [unwired: 9 in, 1 out]
                n183 = Unbundle(w317) -> (w313:string[])
                n184 = Match First String(2:w313, 3:w318) -> (0:w314:i32)  [unwired: 1 out]
                n185 = property on="Test Ring" class="Ring (strict)"("Value"=w314, "Strings []"=w313) -> ()  [unwired: 2 in, 2 out]
                n186 = property on="Test Ring" class="Ring (strict)"("Visible"=TRUE) -> ()  [unwired: 2 in, 2 out]
                n187 = property on="Test Slider" class="Slide (strict)"("Visible"=FALSE) -> ()  [unwired: 2 in, 2 out]
              }
              frame "Exposure Priority  **" {
                n188 = Index Array(array=w325, index=3) -> (element=w326:cluster{string[]})
                n189 = call <vilib>:"NT Read String.vi"("Name"=w328) -> ("String"=w327:string)  [unwired: 9 in, 1 out]
                n190 = Unbundle(w326) -> (w322:string[])
                n191 = Match First String(2:w322, 3:w327) -> (0:w323:i32)  [unwired: 1 out]
                n192 = property on="Test Ring" class="Ring (strict)"("Value"=w323, "Strings []"=w322) -> ()  [unwired: 2 in, 2 out]
                n193 = property on="Test Ring" class="Ring (strict)"("Visible"=TRUE) -> ()  [unwired: 2 in, 2 out]
                n194 = property on="Test Slider" class="Slide (strict)"("Visible"=FALSE) -> ()  [unwired: 2 in, 2 out]
              }
              frame "Color Enable  **" {
                n195 = Index Array(array=w334, index=4) -> (element=w335:cluster{string[]})
                n196 = call <vilib>:"NT Read String.vi"("Name"=w337) -> ("String"=w336:string)  [unwired: 9 in, 1 out]
                n197 = Unbundle(w335) -> (w331:string[])
                n198 = Match First String(2:w331, 3:w336) -> (0:w332:i32)  [unwired: 1 out]
                n199 = property on="Test Ring" class="Ring (strict)"("Value"=w332, "Strings []"=w331) -> ()  [unwired: 2 in, 2 out]
                n200 = property on="Test Ring" class="Ring (strict)"("Visible"=TRUE) -> ()  [unwired: 2 in, 2 out]
                n201 = property on="Test Slider" class="Slide (strict)"("Visible"=FALSE) -> ()  [unwired: 2 in, 2 out]
              }
              frame Default {
                n202 = property on="Test Ring" class="Ring (strict)"("Visible"=FALSE) -> ()  [unwired: 2 in, 2 out]
                n203 = property on="Test Slider" class="Slide (strict)"("Visible"=FALSE) -> ()  [unwired: 2 in, 2 out]
              }
              frame "Brightness  **", "Color Level  **", "Compression  **", "FPS  **", "Sharpness  **" {
                n204 = call <vilib>:"NT Read Number.vi"("Name"=w343) -> ("Numeric"=w342:dbl)  [unwired: 9 in, 1 out]
                n205 = local write "Test Slider"(w342) -> ()
                n206 = property on="Test Slider" class="Slide (strict)"("Visible"=TRUE, "Scale.Maximum"=100.0 ("Scale.Range:Maximum")) -> ()  [unwired: 2 in, 2 out]
                n207 = property on="Test Ring" class="Ring (strict)"("Visible"=FALSE) -> ()  [unwired: 2 in, 2 out]
              }
            }
          }
        }
        n208 = property on="Progress" class="Clust (strict)"("Visible"=FALSE) -> ()  [unwired: 2 in, 2 out]
      }
      event "Test Name": Mouse Enter {
        # "Populate the ring with the list of tests"
        n209 = event-data() -> ()  [unwired: 1 in, 1 out]
        n210 = call <vilib>:"NT Read String Array.vi"("Name"="TestMode/TestList") -> ("String Array"=w351:string[])  [unwired: 9 in, 1 out]
        n211 = Build Array (concatenate)("Select the test to run...", w351) -> (w350:string[])
        n212 = property on="Test Name" class="Ring (strict)"("Strings []"=w350) -> ()  [unwired: 2 in, 2 out]
      }
      event "Test Name": Value Change {
        w353 = FALSE ("Visible")
        # "Tell the robot the test name to run"
        n213 = event-data() -> ("NewVal"=w357:u16)  [unwired: 1 in]
        n214 = property on="Test Name" class="Ring (strict)"() -> ("Strings []"=w358:string[])  [unwired: 2 in, 2 out]
        n215 = local write "Progress"(T9 {"Test Progress"=0, "Test Progress Text"=""} ("Progress")) -> ()
        n216 = Index Array(array=w358, index=w357) -> (element=w356:string)
        n217 = call <vilib>:"NT Write String.vi"("String"=w356, "Name"="TestMode/TestName") -> ()  [unwired: 9 in, 1 out]
        n218 = property on="Progress" class="Clust (strict)"("Visible"=TRUE) -> ()  [unwired: 2 in, 2 out]
        n219 = property on="Motor" class="Clust (strict)"("Visible"=w353) -> ()  [unwired: 2 in, 2 out]
        n220 = property on="Test Slider" class="Slide (strict)"("Visible"=w353) -> ()  [unwired: 2 in, 2 out]
        n221 = property on="On/Off" class="Bool (strict)"("Visible"=w353) -> ()  [unwired: 2 in, 2 out]
        n222 = property on="Rev/Fwd" class="Clust (strict)"("Visible"=w353) -> ()  [unwired: 2 in, 2 out]
        n223 = property on="Test Ring" class="Ring (strict)"("Visible"=w353) -> ()  [unwired: 2 in, 2 out]
      }
      event "Listbox": Double Click {
        # "Shift clears all"
        # "Update symbols on the listbox"
        n224 = event-data() -> ("PlatMods.Shift"=w361:bool, "Row"=w363:i32)  [unwired: 1 in]
        n225 = case shown="True" w361 {
          tunnel: w363 -> [w367 _]
          tunnel: 1 -> [w366 _]
          frame False {
            n226 = property on="Listbox" class="LstBox (strict)"() -> ("Item Symbols"=w365:i32[])  [unwired: 2 in, 2 out]
            n227 = Replace Array Subset(array=w365, new element=w366, index=w367) -> (w364:i32[])
            n228 = property on="Listbox" class="LstBox (strict)"("Item Symbols"=w364) -> ()  [unwired: 2 in, 2 out]
          }
          frame True {
            w368 = 0 ("Top Row")
            n229 = property on="Listbox" class="LstBox (strict)"() -> ("Number of Rows"=w370:u32)  [unwired: 2 in, 2 out]
            n230 = Initialize Array(0, w370) -> (w369:i32[])
            n231 = property on="Listbox" class="LstBox (strict)"("Top Row"=w368, "Value"=w368, "Item Symbols"=w369) -> ()  [unwired: 2 in, 2 out]
          }
        }
      }
      event "Listbox": Key Down {
        # "Update symbols on the listbox\nLeft and right keys check and uncheck"
        n232 = event-data() -> ("VKey"=w374:T25)  [unwired: 1 in]
        n233 = case shown="\"Left\", \"Right\"" w374 {
          selector: w374 -> [w379 _]
          tunnel: eventvkey."Left" ("VKey") -> [w377 _]
          frame "Left", "Right" {
            n234 = Equal?(x=w377, y=w379) -> (x = y?=w378:bool)
            n235 = Select(t=0, s=w378, f=1) -> (s? t:f=w380:i32)
            n236 = property on="Listbox" class="LstBox (strict)"() -> ("Item Symbols"=w383:i32[])  [unwired: 2 in, 2 out]
            n237 = Replace Array Subset(array=w383, new element=w380, index="Listbox") -> (w382:i32[])
            n238 = property on="Listbox" class="LstBox (strict)"("Item Symbols"=w382) -> ()  [unwired: 2 in, 2 out]
          }
          frame Default {
          }
        }
      }
      event "DB Camera Config": Value Change {
        # "Show or hide the cluster of controls, store in ini file"
        n239 = event-data() -> ("NewVal"=w387:bool)  [unwired: 1 in]
        n240 = case shown="False" w387 {
          tunnel: w386 -> [w396 _]
          tunnel: [w389 w407] -> w385
          tunnel: w384 -> [w388 w407]
          frame False {
            w403 = "Camera"
            w406 = FALSE ("Visible")
            n241 = local read "Camera Settings"() -> (w395:T2)
            n242 = Index Array(array=w396) -> (element=w399:cluster{string[]})  [unwired: 1 in]
            n243 = Unbundle(w395) -> ("Frame Rate"=w394:i32, "Compression"=w393:i32, "Size"=w397:u16)
            n244 = Unbundle(w399) -> (w398:string[])
            n245 = Index Array(array=w398, index=w397) -> (element=w392:string)
            n246 = call-poly <vilib>:"Write Key.vi"("section"=w403, "value"=w392, "key"="Size", "refnum"=w388) -> ("refnum out"=w405:T23)  [unwired: 2 in, 5 out]
            n247 = call-poly <vilib>:"Write Key.vi"("section"=w403, "value"=w394, "key"="FrameRate", "refnum"=w405) -> ("refnum out"=w404:T23)  [unwired: 1 in, 6 out]
            n248 = property on="Camera Settings" class="Clust (strict)"("Visible"=w406) -> ()  [unwired: 2 in, 2 out]
            n249 = local write "DB Camera Config"(w406) -> ()
            n250 = call-poly <vilib>:"Write Key.vi"("section"=w403, "value"=w393, "key"="Compression", "refnum"=w404) -> ("refnum out"=w390:T23)  [unwired: 1 in, 6 out]
            n251 = call <vilib>:"Close Config Data.vi"("refnum"=w390) -> ("file path"=w391:path)  [unwired: 2 in, 8 out]
            n252 = call <vilib>:"Open Config Data.vi"("configuration file path"=w391) -> ("refnum"=w389:T23)  [unwired: 8 in, 2 out]
          }
          frame True {
            n253 = property on="Camera Settings" class="Clust (strict)"("Visible"=TRUE) -> ()  [unwired: 2 in, 2 out]
          }
        }
      }
      event "Camera Settings": Value Change {
        # "Update summary string when any elements of DB camera change"
        n254 = event-data() -> ("NewVal"=w420:T2)  [unwired: 1 in]
        n255 = Index Array(array=w416) -> (element=w415:cluster{string[]})  [unwired: 1 in]
        n256 = Unbundle(w420) -> ("Frame Rate"=w411:i32, "Compression"=w410:i32, "Size"=w413:u16)
        n257 = Unbundle(w415) -> (w414:string[])
        n258 = Index Array(array=w414, index=w413) -> (element=w412:string)
        n259 = Format Into String(format string="%s   %dfps   %d%%", w412, w411, w410) -> (resulting string=w417:string)  [unwired: 2 in, 1 out]
        n260 = Build Array(w417) -> (w418:string[])
        n261 = property on="DB Camera Config" class="Bool (strict)"("Strings [4]"=w418) -> ()  [unwired: 2 in, 2 out]
      }
      event "Motor.Enable": Value Change {
        # "When the test mode otor enable helper is set, update that\ntree row item's value"
        n262 = event-data() -> ("NewVal"=w426:bool)  [unwired: 1 in]
        n263 = Unbundle("Motor") -> ("Value"=w425:dbl)  [unwired: 1 out]
        n264 = Select(t=w425, s=w426, f=0.0) -> (s? t:f=w423:dbl)
        n265 = call <vilib>:"NT Write Number.vi"("Numeric"=w423, "Name"=w422) -> ()  [unwired: 9 in, 1 out]
      }
      event "Test Slider": Value Change {
        # "When the test mode slider helper is set, update that\ntree row item's value"
        n266 = event-data() -> ("NewVal"=w429:dbl)  [unwired: 1 in]
        n267 = call <vilib>:"NT Write Number.vi"("Numeric"=w429, "Name"=w430) -> ()  [unwired: 9 in, 1 out]
      }
      event "On/Off": Value Change {
        # "When the test mode on/off helper value is set, update that\ntree row item's value"
        n268 = event-data() -> ("NewVal"=w434:bool)  [unwired: 1 in]
        n269 = Boolean To (0,1)(Boolean=w434) -> (0, 1=w433:i16)
        n270 = call <vilib>:"NT Write Number.vi"("Numeric"=w433, "Name"=w432) -> ()  [unwired: 9 in, 1 out]
      }
      event "Rev/Fwd": Value Change {
        # "When the test mode helper value for relays is set, update that\ntree row item's value"
        n271 = event-data() -> ("NewVal.Forward"=w442:bool, "NewVal.Reverse"=w441:bool)  [unwired: 1 in]
        n272 = Boolean To (0,1)(Boolean=w442) -> (0, 1=w438:i16)
        n273 = Boolean To (0,1)(Boolean=w441) -> (0, 1=w440:i16)
        n274 = Negate(x=w440) -> (-x=w439:i16)
        n275 = Add(x=w438, y=w439) -> (x+y=w437:i16)
        n276 = call <vilib>:"NT Write Number.vi"("Numeric"=w437, "Name"=w436) -> ()  [unwired: 9 in, 1 out]
      }
      event "Test Ring": Value Change {
        # "When a test mode helper value is selected from the ring,\nset the tree item's variable to the string value"
        n277 = event-data() -> ("NewVal"=w446:u16)  [unwired: 1 in]
        n278 = property on="Test Ring" class="Ring (strict)"() -> ("Strings []"=w447:string[])  [unwired: 2 in, 2 out]
        n279 = Index Array(array=w447, index=w446) -> (element=w445:string)
        n280 = call <vilib>:"NT Write String.vi"("String"=w445, "Name"=w444) -> ()  [unwired: 9 in, 1 out]
      }
      event "Rec Mode": Value Change {
        # "Update globals for recording mode and path to read log from.\nClear when logging and let NetworkTables set path for vision to\nuse."
        n281 = event-data() -> ("NewVal"=w457:enum32{"Stop", "Record", "Playback"})  [unwired: 1 in]
        n282 = global write "WPI_DashboardLogging Global.vi" "Logging Filename"(path "") -> ()
        n283 = case shown="\"Playback\"" w457 {
          tunnel: w456 -> [_ w459 w467]
          tunnel: [_ _ w466] -> w453
          tunnel: [_ _ w465] -> _
          tunnel: w451 -> [_ _ w463]
          tunnel: cluster{i32, i32} {-250, 170} -> [_ _ w462]
          tunnel: [_ _ T26 {"Image Size"=TRUE, "Image Type"=TRUE, "Pixel Value"=TRUE, "ROI Information"=TRUE, "Zoom Factor"=FALSE} ("Image Information Shown:All Elements")] -> w449
          tunnel: [_ _ TRUE ("Zoom Factor")] -> w448
          frame Default {
          }
          frame "Stop", "Record" {
            # "Place Window too"
            n284 = invoke class="VI" method="FP.Close"(reference=w459) -> (reference out=w458:refnum<vi>)  [unwired: 2 in, 2 out]
            n285 = invoke class="VI" method="Abort VI"(reference=w458) -> ()  [unwired: 2 in, 3 out]
          }
          frame "Playback" {
            n286 = call "Open Playback Panel.vi"("Offset"=w462, "DB VI Ref"=w463, "Playback in"=w467) -> ("Playback out"=w464:refnum<vi>)  [unwired: 8 in]
            n287 = register-events(w464) -> (reference out=w466:refnum<event-registration>, error out=w465:errorcluster)  [unwired: 2 in]
          }
        }
        n288 = global write "WPI_DashboardLogging Global.vi" "Recording"(w457) -> ()
        n289 = property on="Camera Image" class="ImageControl"("Image Information Shown"=w449, "Image Information Visible"=w448) -> ()  [unwired: 2 in, 2 out]
        n290 = call <vilib>:"WPI_DashboardNT Log FieldName Cache.vi"("Operation"=enum16{"Lookup/Add", "Index", "Clear"}."Clear") -> ()  [unwired: 8 in, 3 out]
      }
      event Panel Close {
        w468 = enum32{"Stop", "Record", "Playback"}."Stop" ("Rec Mode")
        # "Playback window has been closed, abort"
        n291 = event-data() -> ()  [unwired: 1 in, 4 out]
        n292 = local write "Rec Mode"(w468) -> ()
        n293 = global write "WPI_DashboardLogging Global.vi" "Recording"(w468) -> ()
      }
      event Panel Close {
        # "Abort playback window and ourself"
        n294 = event-data() -> ()  [unwired: 1 in, 4 out]
        n295 = invoke class="VI" method="FP.Close"(reference=w473) -> (reference out=w472:refnum<vi>)  [unwired: 2 in, 2 out]
        n296 = invoke class="VI" method="Abort VI"(reference=w472) -> (error out=w471:errorcluster)  [unwired: 2 in, 2 out]
        n297 = invoke class="VI" method="Abort VI"(error in=w471) -> ()  [unwired: 2 in, 3 out]
      }
      event "Vision": Value Change {
        # "Enable/Disable Compression slider.\nHW USB is hard-coded into the camera"
        n298 = event-data() -> ("NewVal"=w479:u16)  [unwired: 1 in]
        n299 = Equal?(x=w479, y=u32 2 ("milliseconds to wait")) -> (x = y?=w477:bool)
        n300 = Select(t=T27."Disabled and Grayed Out" ("Disabled"), s=w477, f=T27."Enabled" ("Disabled")) -> (s? t:f=w474:T27)
        n301 = property on="Compression" class="Slide (strict)"("DisabledEnum"=w474) -> ()  [unwired: 2 in, 2 out]
      }
    }
  }
  n302 = while {
    tunnel: w37 -> [w482]
    i -> [w485]
    stop <- FALSE stop-if-true
    n303 = Wait (ms)(milliseconds to wait=u32 100) -> ()  [unwired: 1 out]
    n304 = case shown="\"Playback\"" "Rec Mode" {
      tunnel: w485 -> [_ _ w500]
      tunnel: [u32 2829099 ("Base Color") u32 11141120 ("Target Color") w489] -> w481
      frame "Stop", Default {
        # "Reset the color, extra updates don't cost much"
      }
      frame "Record" {
      }
      frame "Playback" {
        # "Playback"
        n305 = Quotient & Remainder(x=w500, y=u32 50 ("milliseconds to wait")) -> (x-y*floor(x/y)=w496:u32)  [unwired: 1 out]
        n306 = Divide(x=w496, y=u32 50 ("milliseconds to wait")) -> (x/y=w493:dbl)
        n307 = Multiply(x=6.283185307179586, y=w493) -> (x*y=w498:dbl)
        n308 = Sine(x=w498) -> (sin(x)=w497:dbl)
        n309 = Absolute Value(x=w497) -> (abs(x)=w490:dbl)
        n310 = call "Interpolate RGB Color.vi"("Proportion"=w490, "Target Color"=u32 30976, "Base Color"=u32 2829099) -> ("Result Color"=w489:u32)  [unwired: 8 in]
      }
    }
    n311 = property class="Pane"(reference=w482, "PaneColor"=w481) -> ()  [unwired: 1 in, 2 out]
  }
  n312 = disable-structure shown="Disabled" {
    frame Disabled {
      # "Loop 7. Wait for DS connections"
      n313 = TCP Create Listener(10:u16 1741 ("timeout ms (25000)")) -> (3:w501:refnum<k5>)  [unwired: 4 in, 2 out]
      n314 = while {
        tunnel: w501 -> [w504]
        stop <- FALSE stop-if-true
        n315 = TCP Wait On Listener(11:w504) -> (4:w503:refnum<k5>)  [unwired: 3 in, 4 out]
        n316 = local write "TCP"(w503) -> ()
      }
    }
    frame Enabled {
    }
  }
  n317 = while {
    tunnel: u16 1741 ("timeout ms (25000)") -> [w509]
    stop <- FALSE stop-if-true
    n318 = TCP Create Listener(10:w509) -> (0:w508:errorcluster, 3:w507:refnum<k5>)  [unwired: 4 in, 1 out]
    n319 = case shown="No Error" w508 {
      selector: w508 -> [w510 _]
      tunnel: w507 -> [w511 _]
      frame No Error {
        n320 = while {
          tunnel: w511 -> [w516]
          tunnel: w510 -> [w512]
          stop <- FALSE stop-if-true
          n321 = TCP Wait On Listener(8:w512, 11:w516) -> (0:w514:errorcluster, 4:w515:refnum<k5>)  [unwired: 2 in, 3 out]
          n322 = case shown="Error" w514 {
            frame No Error {
            }
            frame Error {
              n323 = Wait (ms)(milliseconds to wait=u32 100) -> ()  [unwired: 1 out]
            }
          }
          n324 = local write "TCP"(w515) -> ()
        }
      }
      frame Error {
      }
    }
  }
  n325 = property on="On/Off" class="Bool (strict)"("Visible"=w5) -> ()  [unwired: 2 in, 2 out]
  n326 = property on="Motor" class="Clust (strict)"("Visible"=w5) -> ()  [unwired: 2 in, 2 out]
  n327 = property on="Progress" class="Clust (strict)"("Visible"=w5) -> ()  [unwired: 2 in, 2 out]
  n328 = property on="Test Ring" class="Ring (strict)"("Visible"=w5) -> ()  [unwired: 2 in, 2 out]
  n329 = property on="Rev/Fwd" class="Clust (strict)"("Visible"=w5) -> ()  [unwired: 2 in, 2 out]
  n330 = property on="Camera Settings" class="Clust (strict)"("Visible"=w5) -> ()  [unwired: 2 in, 2 out]
  n331 = local write "DB Camera Config"(w5) -> ()
  n332 = global write "WPI_DashboardLogging Global.vi" "Recording"(w31) -> ()
  n333 = local write "Rec Mode"(w31) -> ()
